vi "Fluigent_Pressure_Fluctuation_Final.vi"() -> ()   [LabVIEW 2020]
uses:
  <vilib>/DAQmx/read.llb/DAQmx Read (Analog 1D Wfm NChan NSamp).vi
  <userlib>/Fluigent/Fluigent MFCS/FluigentMFCS_Full.llb/MFCS_EZ Detect.vi
  <userlib>/Fluigent/Fluigent MFCS/FluigentMFCS_Full.llb/MFCS_EZ Initialization.vi
  <vilib>/DAQmx/create/channels.llb/DAQmx Create Channel (AI-Voltage-Basic).vi
  <vilib>/DAQmx/configure/timing.llb/DAQmx Timing (Sample Clock).vi
  <vilib>/Waveform/WDTOps.llb/WDT Get XY Value DBL.vi
  <userlib>/Fluigent/Fluigent MFCS/FluigentMFCS_Full.llb/MFCS_EZ Read All Channels Pressure.vi
  <vilib>/DAQmx/miscellaneous.llb/DAQmx Fill In Error Info.vi
  <userlib>/Fluigent/Fluigent MFCS/FluigentMFCS_Full.llb/MFCS_EZ Close.vi
panel:
  out "Fluigent Waveform":dbl[](graph)
  in  "Sampling Frequency (Hz)":dbl=1000.0
  in  "Voltage Conversion Factor":dbl=100.0 caption="Voltage Conversion Factor (1 V = x mmHg)" format="%0.2f"
  in  "Offset (V)":dbl=0.25 caption="Offset"
  in  "Amplitude (V)":dbl=0.25 caption="Amplitude"
  in  "Phase":dbl
  in  "Reset Signal":bool
  out "Simulated Waveform":dynamicdata(graph)=[{"t0"=timestamp(0.1 s since 1904-01-01), "dt"=0.001, "Y"=[0.25000000000000006, 0.242147310230468, 0.2343023701176717, 0.2264729216703715, 0.21866669160892396, 0.21089138373994237, 0.20315467135356888, 0.19546418965086443, 0.18782752820878634, 0.18025222349019276, 0.17274575140626316, 0.1653155199386772, 0.15796886182883052, 0.15071302734130493, 0.14355517710873186, 0.13650237506511337, 0.1295615814745712, 0.12273964606240723, 0.11604330125525086, 0.10947915553696741, 0.10305368692688174, 0.09677323658675593, 0.09064400256282759, 0.0846720336690871, 0.07886322351782785, 0.07322330470336319, 0.06775784314464714, 0.062472232592385185, 0.057371689306052714, 0.05246124690607748, 0.047745751406263165, 0.043229856431359626, 0.03891801862449626, 0.03481449324901417, 0.030923329989034132, 0.02724836895290811, 0.023793236883495134, 0.020561343579004798, 0.017555878527937163, 0.01477980776144372, 0.012235870926211617, 0.009926578580764317, 0.007854209717842231, 0.006020809515313225, 0.0044281873178278475, 0.0030779148512156407, 0.0019713246713805588, 0.0011095088492300564, 0.0004933178929321103, 0.0001233599085671555, 0.0, 0.0001233599085671555, 0.0004933178929321103, 0.0011095088492300287, 0.001971324671380531, 0.003077914851215585, 0.00442818731782782, 0.006020809515313169, 0.007854209717842203, 0.009926578580764234, 0.01223587092621159, 0.014779807761443636, 0.017555878527937135, 0.020561343579004715, 0.023793236883495106, 0.027248368952908025, 0.030923329989034076, 0.03481449324901409, 0.0389180186244962, 0.04322985643135954, 0.04774575140626311, 0.0524612469060774, 0.05737168930605266, 0.0624722325923851, 0.06775784314464708, 0.0732233047033631, 0.07886322351782779, 0.08467203366908702, 0.09064400256282754, 0.09677323658675585, 0.10305368692688169, 0.10947915553696733, 0.11604330125525081, 0.12273964606240714, 0.12956158147457114, 0.13650237506511326, 0.14355517710873178, 0.1507130273413048, 0.15796886182883046, 0.1653155199386771, 0.17274575140626308, 0.1802522234901926, 0.18782752820878623, 0.1954641896508643, 0.2031546713535688, 0.2108913837399422, 0.21866669160892388, 0.22647292167037134, 0.23430237011767158, 0.24214731023046784], "attributes"=variant("NI_ChannelName"=variant(string "Sine"), "NI_ExpIsRelativeTime"=variant(bool TRUE), "NI_ExpStartTimeStamp"=variant(timestamp timestamp(3697925606.3443184 s since 1904-01-01)), "NI_ExpTimeStamp"=variant(timestamp timestamp(3697925606.4443183 s since 1904-01-01)), "NI_ExpXDimension"=variant(string "t"))}]
  out "Finished":bool=TRUE
  out "Time Elapsed (Min)":cluster{dbl, dbl}(slide)={150.0, 0.013502700000000001} scale=0.0..5.0 scale format="%#_2g"
  out "Dev1 Samples":i32=409
  out "Running":bool
  in  "Signal Frequency (Hz)":dbl=5.0
  in  "Time (min)":dbl(knob)=0.5 min=0.1 max=5.0 step=0.1 scale=0.0..5.0 scale format="%#_2g"
  in  "Session Notes":string[](array[string])=["Sine Wave", "Notes", "test", "1", "1", "junk"]
  out "Analog File Name Fluigent":string="C:\\Users\\kkg5246\\Desktop\\Research\\Fluigent Recordings\\210306_20_33_2506"
  in  "Path for files Fluigent System":path=path "C:/Users/kkg5246/Desktop/Research/Fluigent Recordings"
  in  "Stop":bool
  out "Measured Waveform":waveform(dbl)(graph)={"t0"=timestamp(3697925606.344327 s since 1904-01-01), "dt"=0.001, "Y"=array[409 elements], "attributes"=variant("NI_ChannelName"=variant(string "Dev1/ai0"), "NI_UnitDescription"=variant(string "Volts"))}
  in  "NI Physical Channels":tag="Dev1/ai0"
  # "Wave type"
  # "Notes"
  # "Simulated Signal Parameters"
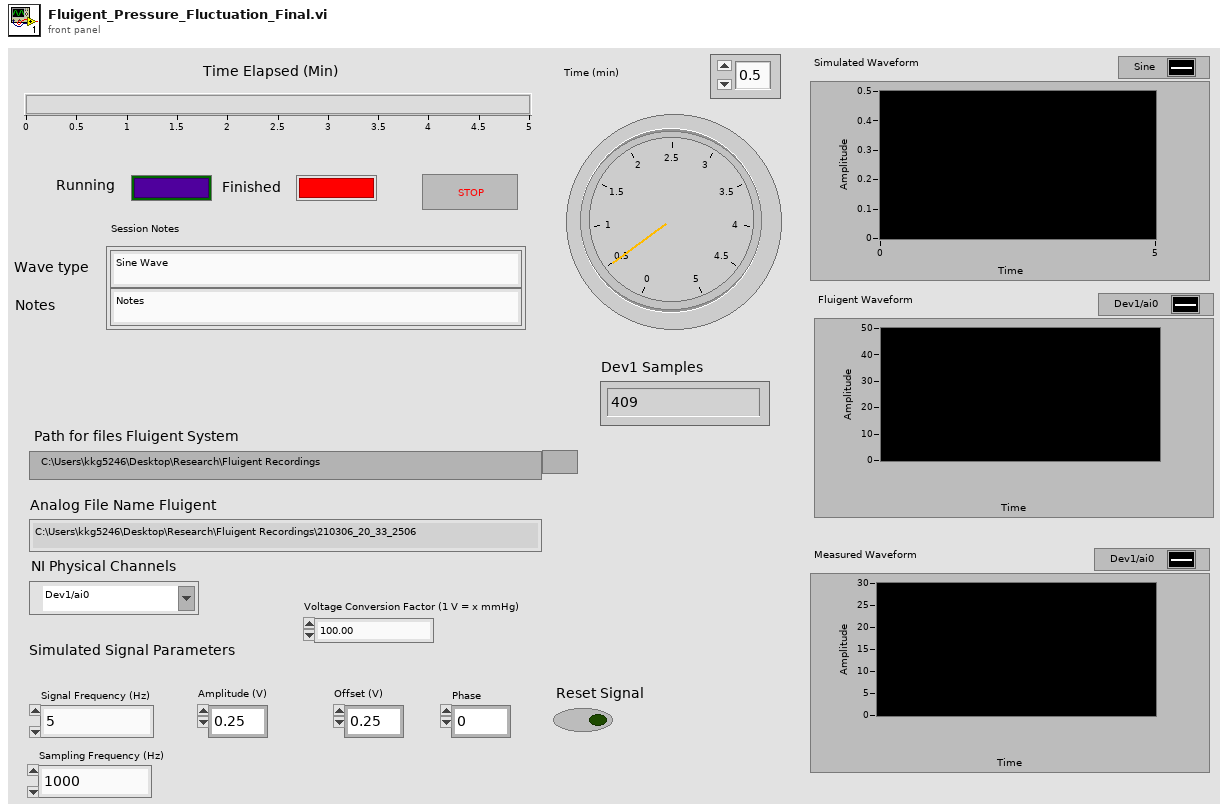
[diagram p1: front panel]
types:
  T1 = enum16{"open", "open or create", "create or replace", "create", "open (read-only)"}
  T2 = typedef "_EZmfcsSN.ctl" = u16
  T3 = typedef "_mfcs_EZ_handle.ctl" = u64
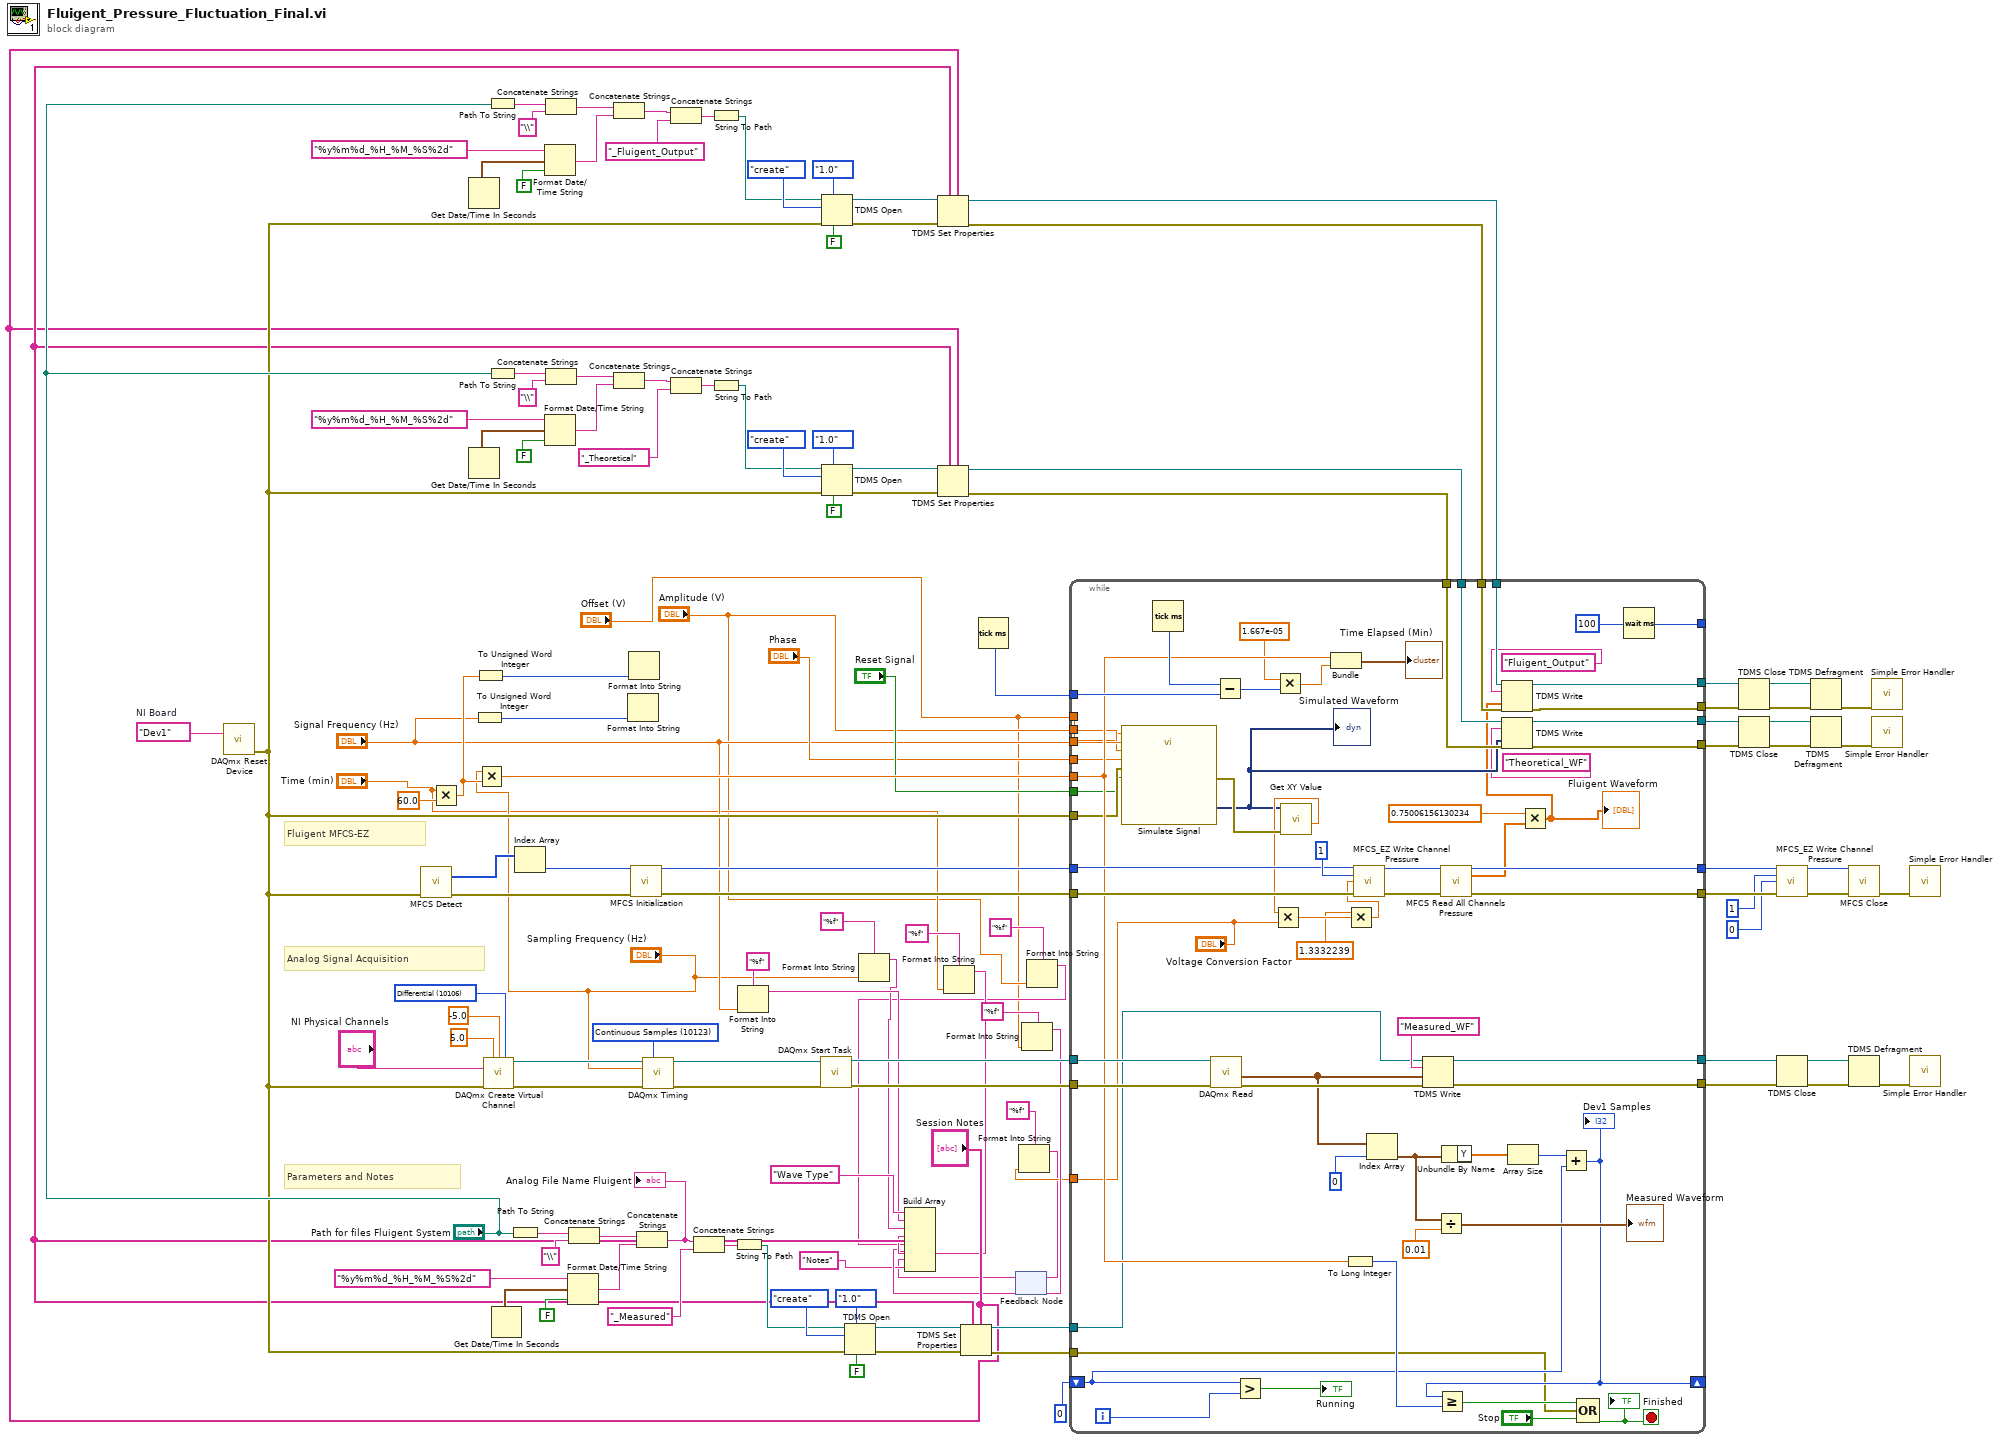
[diagram p0: block diagram]
diagram:
  w87 = tag "Dev1"  # NI Board
  w122 = 10106 items=["default"=-1, "RSE"=10083, "NRSE"=10078, "Differential"=10106, "Pseudodifferential"=12529] ("input terminal configuration")
  w126 = 10123 items=["Finite Samples"=10178, "Continuous Samples"=10123, "Hardware Timed Single Point"=12522] ("sample mode")
  # "Parameters and Notes"
  # "Analog Signal Acquisition"
  # "Fluigent MFCS-EZ"
  n1 = call <vilib>:"DAQmx Reset Device.vi"("device in"=w87) -> ("error out"=w37:errorcluster)  [unwired: 14 in]
  n2 = call-poly <userlib>:"MFCS Detect.vi"("error in (no error)"=w37) -> ("[SN MFCS_EZ]"=w116:T2[], "error out"=w114:errorcluster)  [unwired: 13 in]
  n3 = Multiply(x="Time (min)", y=60.0) -> (x*y=w77:dbl)
  n4 = Get Date/Time In Seconds() -> (seconds since 1Jan1904=w52:timestamp)
  n5 = Get Date/Time In Seconds() -> (seconds since 1Jan1904=w68:timestamp)
  n6 = To Unsigned Word Integer(number="Signal Frequency (Hz)") -> (unsigned 16bit integer=w78:u16)
  n7 = To Unsigned Word Integer(number=w77) -> (unsigned 16bit integer=w76:u16)
  n8 = Multiply(x="Sampling Frequency (Hz)", y=w77) -> (x*y=w85:dbl)
  n9 = call-poly <vilib>:"DAQmx Create Virtual Channel.vi"("maximum value"=5.0, "minimum value"=-5.0, "input terminal configuration"=w122, "physical channels"="NI Physical Channels", "error in"=w37) -> ("task out"=w127:refnum<k21>, "error out"=w125:errorcluster)  [unwired: 4 in, 5 out]
  n10 = Path To String(path="Path for files Fluigent System") -> (string=w43:string)
  n11 = Path To String(path="Path for files Fluigent System") -> (string=w59:string)
  n12 = Get Date/Time In Seconds() -> (seconds since 1Jan1904=w102:timestamp)
  n13 = Path To String(path="Path for files Fluigent System") -> (string=w92:string)
  n14 = Index Array(array=w116) -> (element=w115:T2)  [unwired: 1 in]
  n15 = Format Date/Time String(time format string (%c)="%y%m%d_%H_%M_%S%2d", seconds (now)=w52, UTC format=FALSE) -> (date/time string=w49:string)
  n16 = Format Date/Time String(time format string (%c)="%y%m%d_%H_%M_%S%2d", seconds (now)=w68, UTC format=FALSE) -> (date/time string=w65:string)
  n17 = Concatenate Strings(w43, "\\" ("string")) -> (w50:string)
  n18 = Concatenate Strings(w59, "\\" ("string")) -> (w66:string)
  n19 = Format Date/Time String(time format string (%c)="%y%m%d_%H_%M_%S%2d", seconds (now)=w102, UTC format=FALSE) -> (date/time string=w99:string)
  n20 = Concatenate Strings(w92, "\\" ("string")) -> (w100:string)
  n21 = Concatenate Strings(w50, w49) -> (w40:string)
  n22 = Concatenate Strings(w66, w65) -> (w56:string)
  n23 = Format Into String(w78) -> ()  [unwired: 3 in, 2 out]
  n24 = Format Into String(w76) -> ()  [unwired: 3 in, 2 out]
  n25 = call-poly <userlib>:"MFCS Initialization.vi"("SN MFCS_EZ"=w115, "error in (no error)"=w114) -> ("MFCS_EZ_out"=w110:T3, "error out"=w109:errorcluster)  [unwired: 10 in, 2 out]
  n26 = Concatenate Strings(w100, w99) -> (w72:string)
  "Analog File Name Fluigent" <- w72
  n27 = call-poly <vilib>:"DAQmx Timing.vi"("task/channels in"=w127, "sample mode"=w126, "rate"="Sampling Frequency (Hz)", "error in"=w125) -> ("task out"=w120:refnum<k21>, "error out"=w119:errorcluster)  [unwired: 3 in, 7 out]
  n28 = Concatenate Strings(w40, "_Fluigent_Output" ("string")) -> (w41:string)
  n29 = Concatenate Strings(w56, "_Theoretical" ("string")) -> (w57:string)
  n30 = Concatenate Strings(w72, "_Measured" ("string")) -> (w73:string)
  n31 = String To Path(string=w41) -> (path=w45:path)
  n32 = String To Path(string=w57) -> (path=w61:path)
  n33 = String To Path(string=w73) -> (path=w95:path)
  n34 = Format Into String(format string="%f", "Signal Frequency (Hz)") -> (resulting string=w18:string)  [unwired: 2 in, 1 out]
  n35 = call <vilib>:"DAQmx Start Task.vi"("task/channels in"=w120, "error in"=w119) -> ("task out"=w118:refnum<k21>, "error out"=w117:errorcluster)  [unwired: 12 out]
  n36 = TDMS Open(6:FALSE ("disable buffering? (T)"), 7:enum16{"1.0", "2.0"}."1.0" ("file format version (2.0)"), 8:w37, 10:T1."create" ("operation (0:open)"), 11:w45) -> (0:w44:errorcluster, 3:w42:refnum<k34>)  [unwired: 2 in]
  n37 = TDMS Open(6:FALSE ("disable buffering? (T)"), 7:enum16{"1.0", "2.0"}."1.0" ("file format version (2.0)"), 8:w37, 10:T1."create" ("operation (0:open)"), 11:w61) -> (0:w60:errorcluster, 3:w58:refnum<k34>)  [unwired: 2 in]
  n38 = TDMS Open(6:FALSE ("disable buffering? (T)"), 7:enum16{"1.0", "2.0"}."1.0" ("file format version (2.0)"), 8:w37, 10:T1."create" ("operation (0:open)"), 11:w95) -> (0:w94:errorcluster, 3:w91:refnum<k34>)  [unwired: 2 in]
  n39 = Format Into String(format string="%f", "Sampling Frequency (Hz)") -> (resulting string=w15:string)  [unwired: 2 in, 1 out]
  n40 = Format Into String(format string="%f", "Time (min)") -> (resulting string=w12:string)  [unwired: 2 in, 1 out]
  n41 = Tick Count (ms)() -> (millisecond timer value=w82:u32)
  n42 = feedback #1() -> (w1:string)  [unwired: 1 in]
  n43 = Format Into String(format string="%f", "Offset (V)") -> (resulting string=w6:string)  [unwired: 2 in, 1 out]
  n44 = Format Into String(format string="%f", "Amplitude (V)") -> (resulting string=w9:string)  [unwired: 2 in, 1 out]
  n45 = Build Array("Wave Type", w18, w15, w12, w9, w6, w1, "Notes") -> (w22:string[])
  n46 = TDMS Set Properties(5:"Session Notes", 7:w22, 8:w44, 11:w42) -> (0:w23:errorcluster, 3:w24:refnum<k34>)  [unwired: 4 out]
  n47 = TDMS Set Properties(5:"Session Notes", 7:w22, 8:w60, 11:w58) -> (0:w29:errorcluster, 3:w36:refnum<k34>)  [unwired: 4 out]
  n48 = TDMS Set Properties(5:"Session Notes", 7:w22, 8:w94, 11:w91) -> (0:w90:errorcluster, 3:w88:refnum<k34>)  [unwired: 4 out]
  n49 = while {
    tunnel: w118 -> [w188]
    tunnel: w117 -> [w183]
    tunnel: w110 -> [w184]
    tunnel: w109 -> [w182]
    tunnel: [w152] -> w108
    tunnel: [w181] -> w105
    tunnel: w90 -> [w150]
    tunnel: w88 -> [w151]
    shift-right: [w170] -> _
    shift-left: 0 -> [w171]
    tunnel: w85 -> [w165]
    tunnel: w82 -> [w167]
    tunnel: [w161] -> _
    tunnel: "Signal Frequency (Hz)" -> [w159]
    tunnel: [w155] -> w81
    tunnel: [w154] -> w80
    tunnel: w37 -> [w149]
    tunnel: "Reset Signal" -> [w148]
    tunnel: "Phase" -> [w147]
    tunnel: "Amplitude (V)" -> [w146]
    tunnel: "Offset (V)" -> [w145]
    tunnel: w36 -> [w140]
    tunnel: w29 -> [w139]
    tunnel: [w138] -> w28
    tunnel: [w137] -> w27
    tunnel: [w136] -> w26
    tunnel: [w135] -> w25
    tunnel: w24 -> [w134]
    tunnel: w23 -> [w133]
    tunnel: ["Voltage Conversion Factor"] -> w3
    i -> [w176]
    stop <- w162 stop-if-true
    n50 = call "Simulate Signal"("Offset"=w145, "Reset Signal"=w148, "Frequency"=w159, "Amplitude"=w146, "Phase"=w147, "error in (no error)"=w149) -> ("Sine"=w132:dynamicdata, "error out"=w158:errorcluster)  [unwired: 8 in]
    "Simulated Waveform" <- w132
    n51 = Tick Count (ms)() -> (millisecond timer value=w168:u32)
    n52 = call-poly <vilib>:"DAQmx Read.vi"("task/channels in"=w188, "error in"=w183) -> ("data"=w153:waveform(dbl)[], "error out"=w157:errorcluster)  [unwired: 1 in, 11 out]
    n53 = Subtract(x=w168, y=w167) -> (x-y=w164:u32)
    n54 = Greater?(x=w171, y=w176) -> (0:→"Running":bool)
    n55 = Multiply(x=1.667e-05, y=w164) -> (x*y=w169:dbl)
    n56 = call-poly <vilib>:"Get XY Value.vi"("error in (no error)"=w158, "waveform in"=w132) -> ("Y value"=w142:dbl)  [unwired: 5 in, 4 out]
    n57 = Multiply(x=w142, y="Voltage Conversion Factor") -> (x*y=w144:dbl)
    n58 = Bundle(w165, w169) -> (→"Time Elapsed (Min)":cluster{dbl, dbl})  [unwired: 1 in]
    n59 = To Long Integer(number=w165) -> (32bit integer=w175:i32)
    n60 = Multiply(x=1.3332239, y=w144) -> (x*y=w141:dbl)
    n61 = call <userlib>:"MFCS_EZ Write Channel Pressure.vi"("MFCS_EZ"=w184, "Channel Number (default=1)"=1, "Pressure (mBar)"=w141, "error in (no error)"=w182) -> ("MFCS_EZ out"=w186:T3, "error out"=w187:errorcluster)  [unwired: 10 in]
    n62 = Index Array "Index Array"(array=w153, index=0 ("index (row)")) -> (element=w189:waveform(dbl))
    n63 = TDMS Write(0:w151, 5:"Measured_WF", 9:w153, 11:w157) -> (4:w155:refnum<k34>, 15:w154:errorcluster)  [unwired: 2 in, 2 out]
    n64 = Divide(x=w189, y=0.01) -> (x/y=→"Measured Waveform":waveform(dbl))
    n65 = call-poly <userlib>:"MFCS Read All Channels Pressure.vi"("MFCS_EZ"=w186, "error in (no error)"=w187) -> ("MFCS_EZ out"=w181:T3, "All Channels Pressure"=w180:dbl[], "error out"=w152:errorcluster)  [unwired: 11 in]
    n66 = Unbundle By Name(w189) -> ("Y"=w173:dbl[])
    n67 = TDMS Write(0:w140, 5:"Theoretical_WF", 9:w132, 11:w139) -> (4:w137:refnum<k34>, 15:w138:errorcluster)  [unwired: 2 in, 2 out]
    n68 = Array Size(array=w173) -> (size(s)=w172:i32)
    n69 = Multiply(x=0.75006156130234, y=w180) -> (x*y=w128:dbl[])
    "Fluigent Waveform" <- w128
    n70 = TDMS Write(0:w134, 5:"Fluigent_Output", 9:w128, 11:w133) -> (4:w136:refnum<k34>, 15:w135:errorcluster)  [unwired: 2 in, 2 out]
    n71 = Add(x=w172, y=w171) -> (x+y=w170:i32)
    "Dev1 Samples" <- w170
    n72 = Greater Or Equal?(x=w170, y=w175) -> (x >= y?=w174:bool)
    n73 = Compound Arithmetic op=OR(w174, w150, "Stop") -> (w162:bool)
    "Finished" <- w162
    n74 = Wait (ms)(milliseconds to wait=u32 100) -> (millisecond timer value=w161:u32)
  }
  n75 = Format Into String(format string="%f", w3) -> (resulting string=w2:string)  [unwired: 2 in, 1 out]
  n76 = feedback-in #1(w2) -> ()
  n77 = TDMS Close(8:w25, 11:w26) -> (0:w35:errorcluster, 3:w33:path)
  n78 = TDMS Close(8:w28, 11:w27) -> (0:w32:errorcluster, 3:w30:path)
  n79 = call <userlib>:"MFCS_EZ Write Channel Pressure.vi"("MFCS_EZ"=w105, "Channel Number (default=1)"=1, "Pressure (mBar)"=0, "error in (no error)"=w108) -> ("MFCS_EZ out"=w111:T3, "error out"=w112:errorcluster)  [unwired: 10 in]
  n80 = TDMS Close(8:w80, 11:w81) -> (0:w89:errorcluster, 3:w83:path)
  n81 = TDMS Defragment(4:w35, 7:w33) -> (0:w34:errorcluster)
  n82 = TDMS Defragment(4:w32, 7:w30) -> (0:w31:errorcluster)
  n83 = call-poly <userlib>:"MFCS Close.vi"("MFCS_EZ"=w111, "error in (no error)"=w112) -> ("error out"=w113:errorcluster)  [unwired: 13 in]
  n84 = TDMS Defragment(4:w89, 7:w83) -> (0:w84:errorcluster)
  n85 = call <vilib>:"Simple Error Handler.vi"("error in (no error)"=w34) -> ()  [unwired: 4 in, 5 out]
  n86 = call <vilib>:"Simple Error Handler.vi"("error in (no error)"=w31) -> ()  [unwired: 4 in, 5 out]
  n87 = call <vilib>:"Simple Error Handler.vi"("error in (no error)"=w113) -> ()  [unwired: 4 in, 5 out]
  n88 = call <vilib>:"Simple Error Handler.vi"("error in (no error)"=w84) -> ()  [unwired: 4 in, 5 out]
